vi "vit 4th problem.vi"() -> ()   [LabVIEW 2020]
uses:
  <vilib>/numeric/Random Number (Range) U64.vi
  <vilib>/numeric/sub_Random U32.vi
panel:
  in  "stop":bool
  out "Error":string
  in  "Input":dbl
  out "LED":bool
  out "o/p":dbl
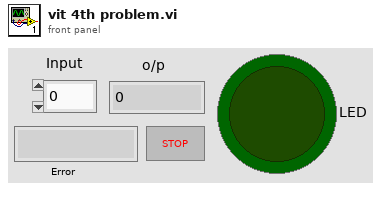
[diagram p1: front panel]
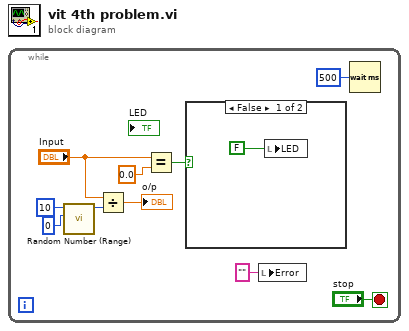
[diagram p0: block diagram]
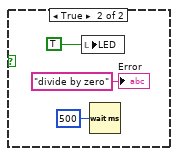
[diagram p2: hidden frame]
diagram:
  n1 = while {
    stop <- "stop" stop-if-true
    n2 = call-poly <vilib>:"Random Number (Range).vi"("lower bound (0)"=u64 0, "upper bound (100)"=u64 10) -> ("number"=w9:u64)  [unwired: 9 in]
    n3 = Divide(x="Input", y=w9) -> (x/y=→"o/p":dbl)
    n4 = Equal?(x="Input", y=0.0) -> (x = y?=w10:bool)
    n5 = case shown="False" w10 {
      frame False {
        n6 = local write "LED"(FALSE ("Boolean")) -> ()
      }
      frame True {
        n7 = local write "LED"(TRUE ("Boolean")) -> ()
        n8 = Wait (ms)(milliseconds to wait=u32 500 ("millisecond timer value")) -> ()  [unwired: 1 out]
        "Error" <- "divide by zero"
      }
    }
    n9 = local write "Error"("" ("Error")) -> ()
    n10 = Wait (ms)(milliseconds to wait=u32 500 ("millisecond timer value")) -> ()  [unwired: 1 out]
  }
